vi "PH_DIM.add Long Integer Service.vi"(0 "i ref in":refnum<vi>, 1 "Service Name":string="N/A", 2 "Number":i32, 5 "error in (no error)":errorcluster) -> (14 "i ref out":refnum<vi>, 17 "Service ID":i32, 19 "error out":errorcluster)   [LabVIEW 2014, in "PH_Common.lvlib"]
doc: "This VI publishes a double number opening a service \"<instancename>_ServiceName\", if no error comes in, and the ServiceName is not N/A. For further use, the Service ID is given out (it is \"-1\" if the service has not been added)."
uses:
  PH_Common.lvlib
  lib.lib/DimLVEvent/LVDimInterface/LVDimInterface.lvlib
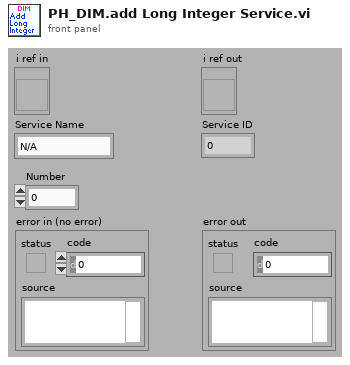
[diagram p1: front panel]
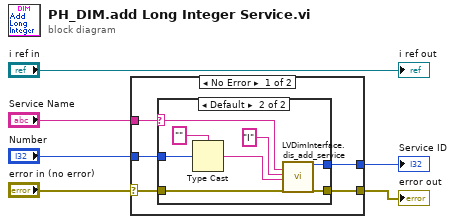
[diagram p0: block diagram]
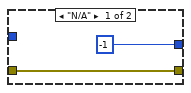
[diagram p2: hidden frame]
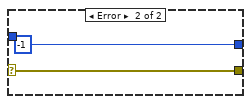
[diagram p3: hidden frame]
diagram:
  n1 = case shown="No Error" "error in (no error)" {
    selector: "error in (no error)" -> [w9 w23]
    tunnel: [w11 -1 ("my_serviceID")] -> w6
    tunnel: [w10 w23] -> w5
    tunnel: "Number" -> [w8 _]
    tunnel: "Service Name" -> [w7 _]
    frame No Error {
      n2 = case shown="Default" w7 {
        selector: w7 -> [_ w15]
        tunnel: [-1 ("my_serviceID") w17] -> w11
        tunnel: [w13 w18] -> w10
        tunnel: w9 -> [w13 w19]
        tunnel: w8 -> [_ w16]
        frame "N/A" {
        }
        frame Default {
          n3 = Type Cast(type="", x=w16) -> (*(type *) &x=w21:string)
          n4 = call "LVDimInterface.dis_add_service.vi"("serviceName"=w15, "typeDescriptor"="I", "data"=w21, "error in (no error)"=w19) -> ("my_serviceID"=w17:i32, "error out"=w18:errorcluster)  [unwired: 14 in]
        }
      }
    }
    frame Error {
    }
  }
  "Service ID" <- w6
  "error out" <- w5
  "i ref out" <- "i ref in"
